vi "Extract Signal Bits from Byte Array.vi"(7 "Payload":u8[](array[numeric]), 10 "Bit Length":i32, 11 "Start Bit":i32) -> (3 "Signal Bits":bool[](array[boolean]))   [LabVIEW 2023, in "CAN Frame.lvclass"]
uses:
  CAN Frame.lvclass
  CAN Frame.lvclass/CAN Frame.ctl
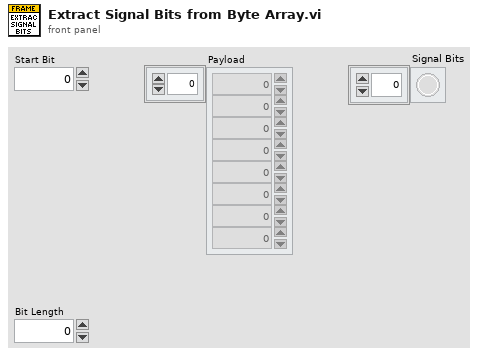
[diagram p1: front panel]
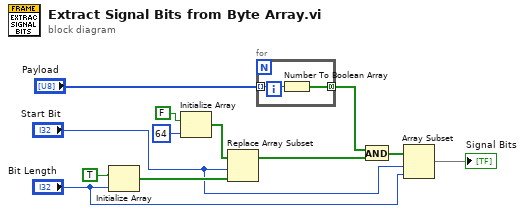
[diagram p0: block diagram]
diagram:
  n1 = Initialize Array(TRUE ("element"), "Bit Length") -> (w8:bool[])
  n2 = Initialize Array(FALSE ("element"), 64 ("dimension size")) -> (w9:bool[])
  n3 = Replace Array Subset(array=w9, new element=w8, index="Start Bit") -> (w6:bool[])
  n4 = for {
    tunnel: "Payload" -> [w14] mode=indexing
    tunnel: [w13] -> w5 mode=concatenating
    n5 = Number To Boolean Array(number=w14) -> (Boolean array=w13:bool[])
  }
  n6 = And(x=w5, y=w6) -> (x .and. y?=w4:bool[])
  n7 = Array Subset(array=w4, index="Start Bit", length="Bit Length") -> (→"Signal Bits":bool[])
